vi "Begin.vi"(8 "error in":errorcluster) -> (0 "error out":errorcluster)   [LabVIEW 2019]
doc: "Called before other user functions, this VI is expected to open initial I/O refnums, load in file data, and do all program initialization. Notice that the <B>error out</B> terminal is simply used for data flow. Wiring it to other structures or subVIs ensures that this VI runs first."
uses:
  <vilib>/Rock Robotics/WPI/DriverStation/WPI_DriverStationRobotMode2.ctl
  <vilib>/Rock Robotics/WPI/Joystick/WPI_JoystickDeviceEnum.ctl
  Robot Global Data.vi
  Joystick_Globals.vi
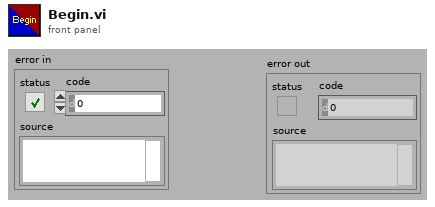
[diagram p1: front panel]
types:
  T1 = typedef "WPI_JoystickDeviceEnum.ctl" = enum16{"USB 0", "USB 1", "USB 2", "USB 3", "USB 4", "USB 5"}
  T2 = typedef "WPI_DriverStationRobotMode2.ctl" = enum16{"Autonomous Disabled", "Autonomous Enabled", "Teleop Disabled", "Teleop Enabled", "Disconnected", "Finish", "Test Disabled", "Test Enabled", "Emergency Stopped"}
  T3 = typedef "WPI_CompressorDevRef.ctl" = cluster{"DevStatus":errorcluster, "Pneumatics Control Module":u8}
  T4 = typedef "WPI_JoystickDevRef.ctl" = cluster{"Device":T1}
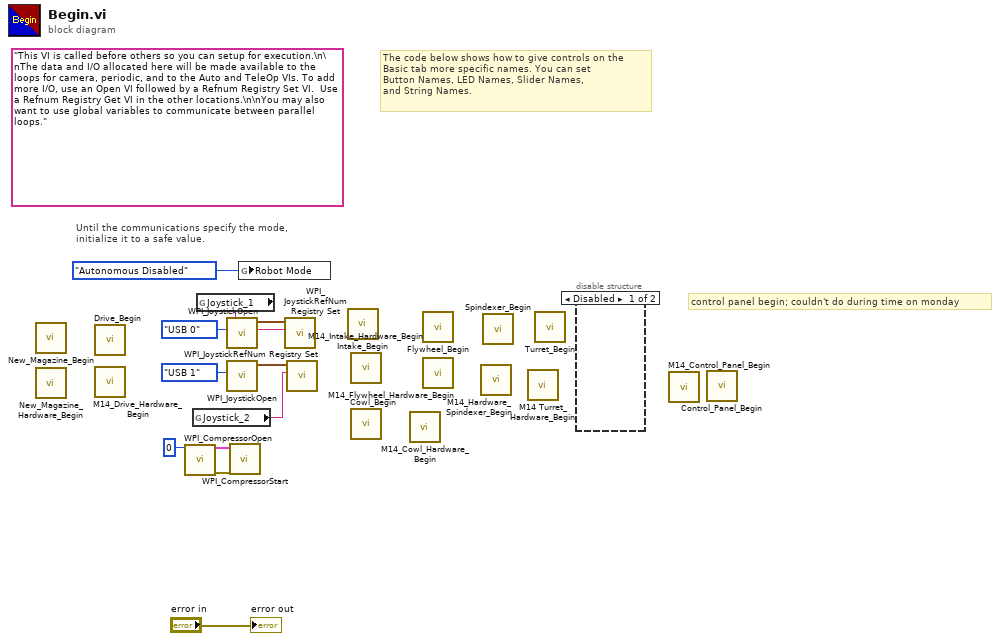
[diagram p0: block diagram]
diagram:
  (unwired) "This VI is called before others so you can setup for execution.\n\nThe data and I/O allocated here will be made available to the loops for camera, periodic, and to the Auto and TeleOp VIs. To add more I/O, use an Open VI followed by a Refnum Registry Set VI.  Use a Refnum Registry Get VI in the other locations.\n\nYou may also want to use global variables to communicate between parallel loops."
  # "control panel begin; couldn't do during time on monday"
  # "The code below shows how to give controls on the\nBasic tab more specific names. You can set\nButton Names, LED Names, Slider Names,\nand String Names."
  # "Until the communications specify the mode,\ninitialize it to a safe value."
  n1 = call "New_Magazine_Begin.vi"() -> ()  [unwired: 12 in]
  n2 = call "New_Magazine_Hardware_Begin.vi"() -> ()  [unwired: 12 in]
  n3 = call "Drive_Begin.vi"() -> ()  [unwired: 12 in]
  n4 = call "M14_Drive_Hardware_Begin.vi"() -> ()  [unwired: 12 in]
  n5 = call <vilib>:"WPI_CompressorOpen.vi"("Pneumatics Control Module (0)"=u8 0) -> ("CompressorDevRef"=w1:T3, "error out"=w2:errorcluster)  [unwired: 13 in]
  n6 = global read "Joystick_Globals.vi" "Joystick_2"() -> (w4:string)
  n7 = global read "Joystick_Globals.vi" "Joystick_1"() -> (w5:string)
  n8 = call <vilib>:"WPI_JoystickOpen.vi"("JoystickDevice"=WPI_JoystickDeviceEnum."USB 0") -> ("JoystickDevRef"=w7:T4)  [unwired: 10 in]
  n9 = call <vilib>:"WPI_JoystickOpen.vi"("JoystickDevice"=WPI_JoystickDeviceEnum."USB 1") -> ("JoystickDevRef"=w6:T4)  [unwired: 10 in]
  n10 = call <vilib>:"WPI_CompressorStart.vi"("error in (no error)"=w2, "CompressorDevRef"=w1) -> ()  [unwired: 8 in, 2 out]
  n11 = global write "Robot Global Data.vi" "Robot Mode"(WPI_DriverStationRobotMode2."Autonomous Disabled" ("Robot Mode")) -> ()
  n12 = call <vilib>:"WPI_JoystickRefNum Registry Set.vi"("refnum name"=w5, "JoystickDevRef"=w7) -> ()  [unwired: 8 in, 2 out]
  n13 = call <vilib>:"WPI_JoystickRefNum Registry Set.vi"("refnum name"=w4, "JoystickDevRef"=w6) -> ()  [unwired: 8 in, 2 out]
  n14 = call "Intake_Begin.vi"() -> ()  [unwired: 12 in]
  n15 = call "M14_Intake_Hardware_Begin.vi"() -> ()  [unwired: 12 in]
  n16 = call "Cowl_Begin.vi"() -> ()  [unwired: 12 in]
  n17 = call "M14_Cowl_Hardware_Begin.vi"() -> ()  [unwired: 12 in]
  n18 = call "Flywheel_Begin.vi"() -> ()  [unwired: 12 in]
  n19 = call "M14_Flywheel_Hardware_Begin.vi"() -> ()  [unwired: 12 in]
  n20 = call "M14_Hardware_Spindexer_Begin.vi"() -> ()  [unwired: 12 in]
  n21 = call "Spindexer_Begin.vi"() -> ()  [unwired: 12 in]
  n22 = call "M14 Turret_Hardware_Begin.vi"() -> ()  [unwired: 12 in]
  n23 = call "Turret_Begin.vi"() -> ()  [unwired: 12 in]
  n24 = disable-structure shown="Disabled" {
    frame Disabled {
    }
    frame Enabled {
    }
  }
  n25 = call "M14_Control_Panel_Begin.vi"() -> ()  [unwired: 12 in]
  n26 = call "Control_Panel_Begin.vi"() -> ()  [unwired: 12 in]
  "error out" <- "error in"
